vi "create rxtx.vi"(8 "error in (no error)":errorcluster, 9 "qeue name":string, 10 "remote IP":string, 11 "Server in":refnum<class "Server.lvclass">) -> (0 "error out":errorcluster, 3 "Server out":refnum<class "Server.lvclass">)   [LabVIEW 2018, in "Server.lvclass"]
uses:
  Server.lvclass
  Server.lvclass/Server.ctl
  RxTx/CCS_RxTx.lvclass
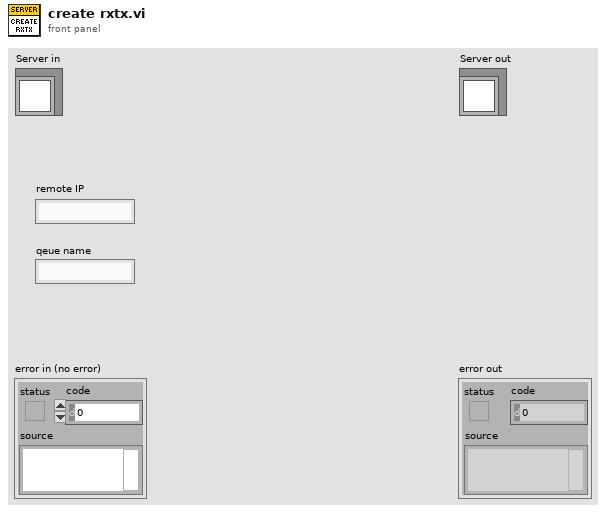
[diagram p1: front panel]
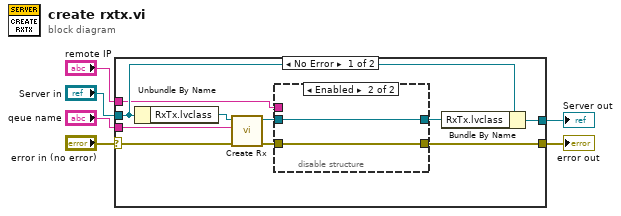
[diagram p0: block diagram]
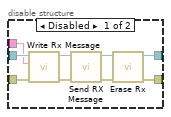
[diagram p2: hidden frame]
diagram:
  n1 = case shown="No Error" "error in (no error)" {
    selector: "error in (no error)" -> [w12 w29]
    tunnel: [w11 w29] -> w5
    tunnel: [w13 w28] -> w3
    tunnel: "Server in" -> [w15 w28]
    tunnel: "remote IP" -> [w9 _]
    tunnel: "qeue name" -> [w10 _]
    frame No Error {
      n2 = Unbundle By Name(w15) -> ("RxTx.lvclass"=w16:refnum<class "CCS_RxTx.lvclass">)
      n3 = call "Create Rx.vi"("error in (no error)"=w12, "Reader Name"=w10, "RxTx in"=w16) -> ("error out"=w7:errorcluster, "RxTx out"=w8:refnum<class "CCS_RxTx.lvclass">)  [unwired: 7 in]
      n4 = disable-structure shown="Enabled" {
        disable-tunnel: w7 -> [w18 w26]
        disable-tunnel: w8 -> [w21 w27]
        disable-tunnel: [w23 w27] -> w14
        disable-tunnel: [w22 w26] -> w11
        disable-tunnel: w9 -> [w17 _]
        frame Disabled {
          n5 = call "Write Rx Message.vi"("error in (no error)"=w18, "Rx Message"=w17, "RxTx in"=w21) -> ("error out"=w19:errorcluster, "RxTx out"=w20:refnum<class "CCS_RxTx.lvclass">)  [unwired: 7 in]
          n6 = call "Send RX Message.vi"("error in (no error)"=w19, "RxTx in"=w20) -> ("error out"=w25:errorcluster, "RxTx out"=w24:refnum<class "CCS_RxTx.lvclass">)  [unwired: 8 in]
          n7 = call "Erase Rx.vi"("error in (no error)"=w25, "RxTx in"=w24) -> ("error out"=w22:errorcluster, "RxTx out"=w23:refnum<class "CCS_RxTx.lvclass">)  [unwired: 8 in]
        }
        frame Enabled {
        }
      }
      n8 = Bundle By Name(cluster=w15, "RxTx.lvclass"=w14) -> (w13:refnum<class "Server.lvclass">)
    }
    frame Error {
    }
  }
  "error out" <- w5
  "Server out" <- w3
